vi "Load PIC and XML.vi"(4 "selected path":path) -> (2 "toChanger":T1(array[cluster]), 3 "vi refnum":refnum<vi>)   [LabVIEW 2019]
uses:
  <vilib>/Utility/config.llb/Read Key (Path).vi
  <vilib>/Utility/config.llb/NI_LVConfig.lvlib
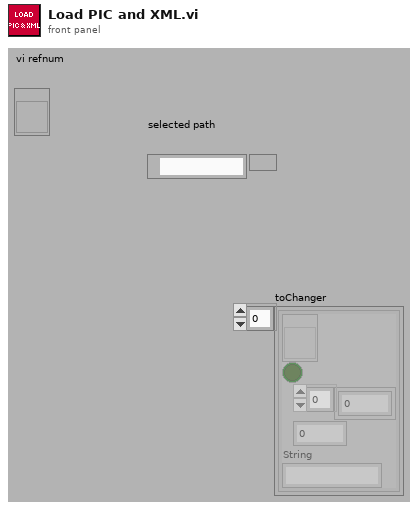
[diagram p1: front panel]
types:
  T1 = cluster{refnum<vi>, bool, i32[], i32, "String":string}[]
  T2 = typedef "NI_LVConfig.lvlib/Config Data RefNum.ctl" = refnum<k1>
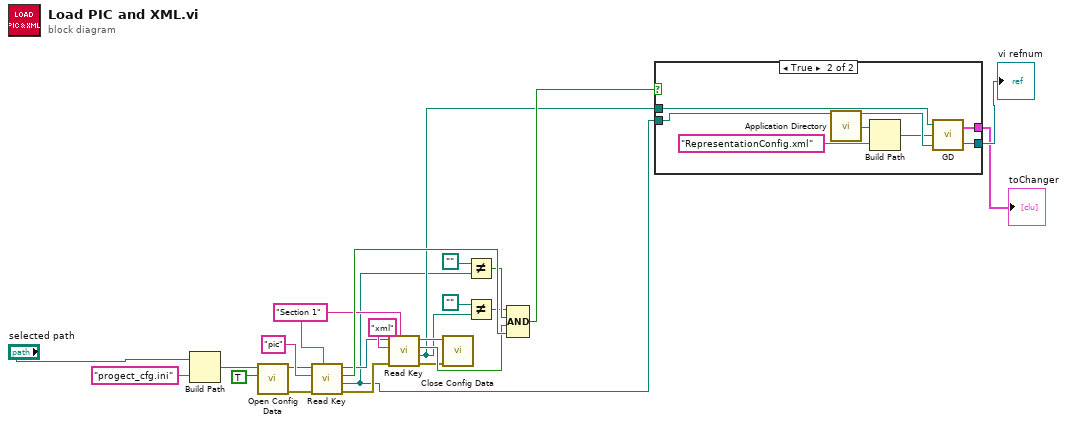
[diagram p0: block diagram]
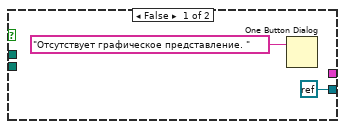
[diagram p2: hidden frame]
diagram:
  w17 = "Section 1" ("section")
  n1 = Build Path(base path="selected path", name or relative path="progect_cfg.ini") -> (appended path=w7:path)
  n2 = call <vilib>:"Open Config Data.vi"("create file if necessary (T)"=TRUE, "configuration file path"=w7) -> ("error out"=w9:errorcluster, "refnum"=w10:T2)  [unwired: 7 in, 1 out]
  n3 = call-poly <vilib>:"Read Key.vi"("section"=w17, "error in (no error)"=w9, "key"="pic", "refnum"=w10) -> ("error out"=w13:errorcluster, "value"=w3:path, "found?"=w23:bool, "refnum out"=w12:T2)  [unwired: 4 in]
  n4 = call-poly <vilib>:"Read Key.vi"("section"=w17, "error in (no error)"=w13, "key"="xml", "refnum"=w12) -> ("error out"=w15:errorcluster, "value"=w4:path, "found?"=w22:bool, "refnum out"=w14:T2)  [unwired: 4 in]
  n5 = call <vilib>:"Close Config Data.vi"("error in (no error)"=w15, "refnum"=w14) -> ()  [unwired: 8 in, 2 out]
  n6 = Not Equal?(x=path "", y=w3) -> (x != y?=w21:bool)
  n7 = Not Equal?(x=path "", y=w4) -> (x != y?=w20:bool)
  n8 = Compound Arithmetic op=AND(w20, w21, w22, w23) -> (w24:bool)
  n9 = case shown="True" w24 {
    tunnel: w3 -> [_ w30]
    tunnel: w4 -> [_ w33]
    tunnel: [refnum<k0> refnum w32] -> w2
    tunnel: [_ w31] -> w1
    frame False {
      n10 = One Button Dialog(message="Отсутствует графическое представление. ") -> ()  [unwired: 1 in, 1 out]
    }
    frame True {
      n11 = call <vilib>:"Application Directory.vi"() -> ("Application Directory"=w28:path)
      n12 = Build Path(base path=w28, name or relative path="RepresentationConfig.xml") -> (appended path=w27:path)
      n13 = call "GD.vi"("BMP File Path"=w30, "XML indicator's config Path"=w27, "XML File Path"=w33) -> ("vi refnum"=w32:refnum<vi>, "toChanger"=w31:T1)
    }
  }
  "vi refnum" <- w2
  "toChanger" <- w1
